vi "N6701A_SetVoltage.vi"(8 "error in (no error)":errorcluster, 9 "Level  (0.0 volts)":dbl format="%^.3e", 10 "Channel Name (1)":string="1", 11 "VISA resource name":refnum<visa-resource-name>) -> (0 "error out":errorcluster)   [LabVIEW 2015]
doc: "This VI will set the Voltage to include negative values"
uses:
  <instrlib>/Agilent N6700 Series/Agilent N6700 Series.lvlib
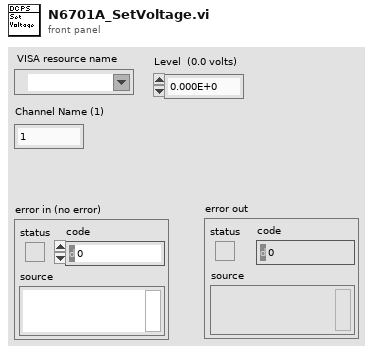
[diagram p1: front panel]
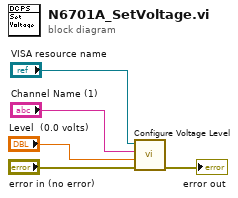
[diagram p0: block diagram]
diagram:
  n1 = call <instrlib>:"Configure Voltage Level.vi"("error in (no error)"="error in (no error)", "Level  (0.0 volts)"="Level  (0.0 volts)", "Channel Name (1)"="Channel Name (1)", "VISA resource name"="VISA resource name") -> ("error out"=→"error out":errorcluster)  [unwired: 6 in, 1 out]
